vi "Release Waiting Procs.vi"(8 "error in (no error)":errorcluster, 11 "Notifiers":refnum<queue>[](array[refnum])) -> (0 "Error Out":errorcluster, 3 "Notifiers Out":refnum<queue>[](array[refnum]))   [LabVIEW 2020]
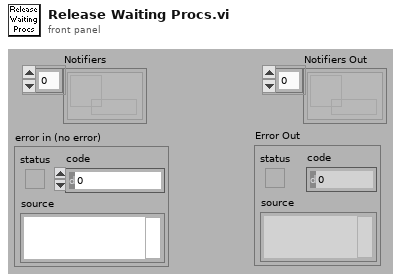
[diagram p1: front panel]
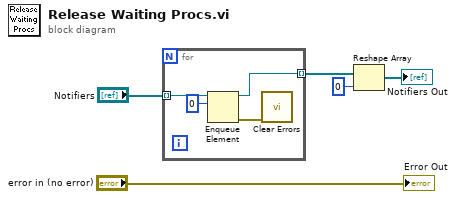
[diagram p0: block diagram]
diagram:
  n1 = for {
    tunnel: "Notifiers" -> [w9] mode=indexing
    tunnel: [w7] -> w4 mode=indexing
    n2 = Enqueue Element(queue=w9, element=0) -> (queue out=w7:refnum<queue>, error out=w6:errorcluster)  [unwired: 1 in, 2 out]
    n3 = call "Clear Errors.vi"("error in (no error)"=w6) -> ()  [unwired: 5 in, 2 out]
  }
  n4 = Reshape Array(w4, 0 ("dimension size")) -> (→"Notifiers Out":refnum<queue>[])
  "Error Out" <- "error in (no error)"
